vi "Sick Loop.vi"() -> ()   [LabVIEW 2009]
uses:
  <vilib>/Platform/TimedLoop/XDataNode/XDataNode.xnode
  <vilib>/Platform/TimedLoop/XDataNode/loadlvalarms.vi
  <vilib>/Platform/TimedLoop/XDataNode/timing_clust.ctl
  <vilib>/Platform/TimedLoop/XDataNode/nitl_modes.ctl
  <vilib>/Platform/TimedLoop/XDataNode/wakeup.ctl
  TypeDefs/Sensor TypeDefs/FPGA Main ref.ctl
  <vilib>/userDefined/High Color/nirio_resource_hc.ctl
  <vilib>/rvi/interface/nirviOpenFPGA/nirviOpenFPGA.xnode
  FPGA Bitfiles/Q_IGVC_2010.lvproj_FPGA Target_FPGA_MAIN.vi.lvbitx
  <vilib>/FPGAPlugInAG/cRIO-9113/nirviIntfOpen_cRIO-9113.vi
  Functional Global Variables/Actions for FG's.ctl
  UI Comm/Watchdog Dish Labels.ctl
  <vilib>/Platform/TimedLoop/XDataNode/XDNodeRunTimeDep.lvlib
panel:
  in  "SICK Init Complete":bool
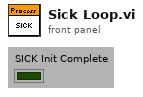
[diagram p1: front panel]
types:
  T1 = typedef "FPGA Main ref.ctl" = refnum<k20>
  T2 = typedef "nirio_resource_hc.ctl" = tag
  T3 = cluster{"signature":u8[], "vi signatures match":bool, "signature register address":u32, "reset register address":u32, "control register address":u32, "interrupt base address":u32, "Bitstream Version":u32, "DMA Configuration":cluster{"Name":string, "Depth":u32, "Write? (Deprecated:Use Implementation)":bool, "Physical Channel":u32, "Base Address":u32, "Data Width":u32, "Data Type":enum32{"Boolean", "I8", "I16", "I32", "I64", "U8", "U16", "U32", "U64", "FXP"}, "FXP Properties":variant, "Write Window Address":u32, "Implementation":enum16{"niFpgaTargetToHost", "niFpgaHostToTarget", "niFpgaPeerToPeerWriter", "niFpgaPeerToPeerReader", "niCoreTargetToHost", "niCoreHostToTarget"}, "Control Set":u32}[], "run when loaded?":bool, "reset register size in bits":u32, "compilation results xml":string}
  T4 = typedef "XDNodeRunTimeDep.lvlib/timing_clust.ctl" = cluster{"Expected End [f-1]":u64, "Actual End [f-1]":u64, "Finished Late? [f-1]":bool, "Expected End [i-1]":u64, "Actual End [i-1]":u64, "Finished Late? [i-1]":bool, "Expected Start [i]":u64, "Actual Start [i]":u64, "Expected Start [f]":u64, "Actual Start [f]":u64, "Source Name":string, "Structure Name":string, "Period":i64, "Deadline":i64, "Offset":i64, "Start":i64, "Priority":i32, "Timeout":i32, "Mode":T5, "Wakeup Reason":T6, "Error":errorcluster, "Source Type":string, "Secondary Source Type":string, "Global End Time":u64, "Global Start Time":u64, "Frame Duration":u64, "Iteration Duration":u64, "Assigned CPU":i32, "I/O Scan Engine Mode":u32}
  T5 = typedef "XDNodeRunTimeDep.lvlib/nitl_modes.ctl" = enum32{"No Change", "Process missed periods, maintain original phase", "Discard missed periods, maintain original phase", "Process missed periods, ignore original phase", "Discard missed periods, ignore original phase"}
  T6 = typedef "XDNodeRunTimeDep.lvlib/wakeup.ctl" = enum32{"Normal", "Aborted", "Asynchronous wakeup", "Timing source error", "Timed loop error", "Timeout"}
  T7 = typedef "SICK Array.ctl" = u16[]
  T8 = typedef "Actions for FG's.ctl" = enum16{"Read", "Write"}
  T9 = typedef "Watchdog Dish Labels.ctl" = enum16{"GPS", "SICK", "Compass", "Cameras", "Motor Controller", "Debug", "RC Receiver"}
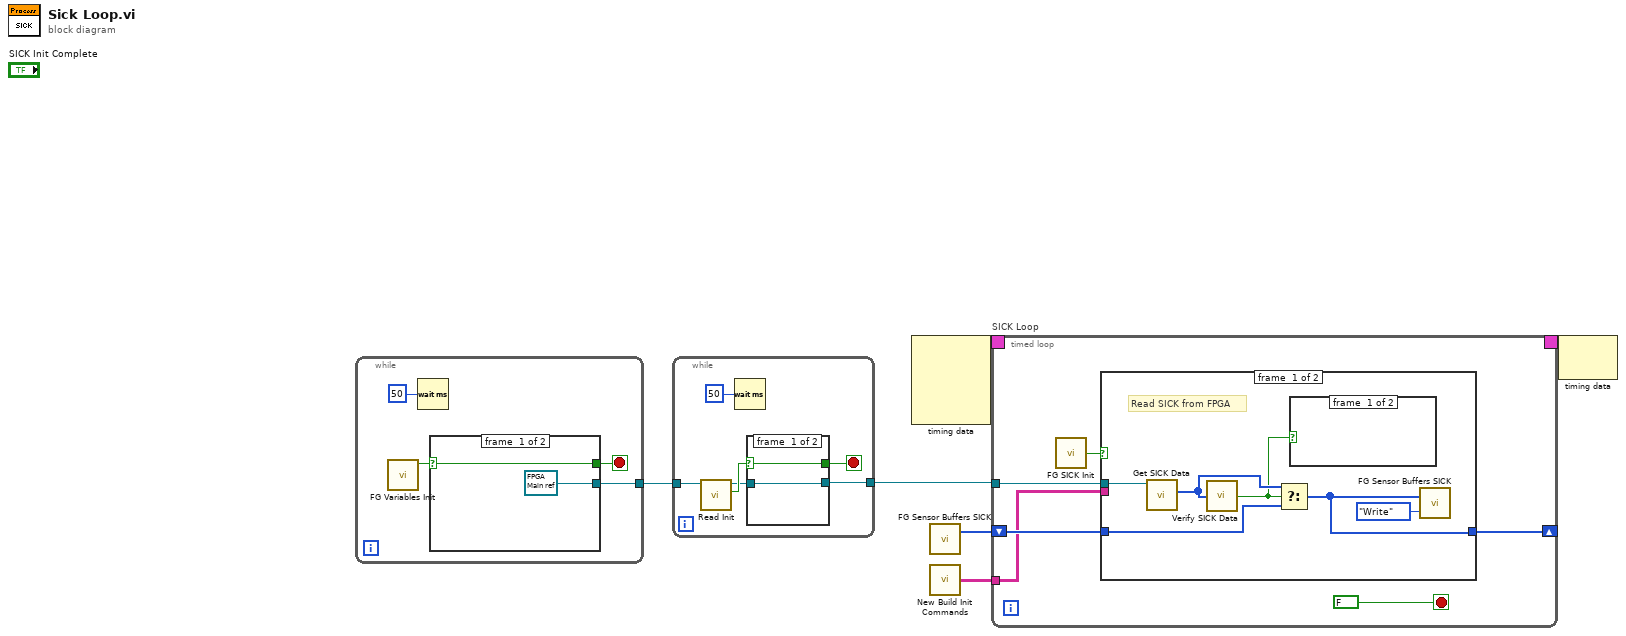
[diagram p0: block diagram]
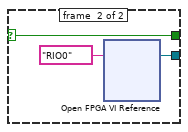
[diagram p2: hidden frame]
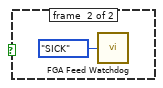
[diagram p4: hidden frame]
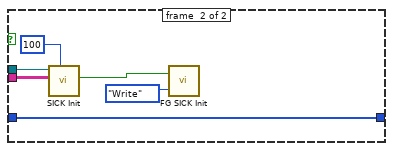
[diagram p5: hidden frame]
diagram:
  n1 = while {
    tunnel: [w8] -> w1
    stop <- w9 stop-if-true
    n2 = call "FG Variables Init.vi"() -> ("Variables Init out"=w10:bool)  [unwired: 11 in]
    n3 = Wait (ms)(milliseconds to wait=u32 50) -> ()  [unwired: 1 out]
    n4 = case shown="True" w10 {
      selector: w10 -> [w12 w15]
      tunnel: [w12 w15] -> w9
      tunnel: [T1 refnum ("FPGA VI Reference out") w13] -> w8
      frame #0 {
      }
      frame #1 {
        n5 = xnode "Open FPGA VI Reference"("resource name"=T2 "RIO0") -> ("FPGA VI Reference Out"=w13:refnum<k20>)  [unwired: 1 in, 1 out]
      }
    }
  }
  n6 = while {
    tunnel: [w31] -> w2
    tunnel: w1 -> [w29]
    stop <- w32 stop-if-true
    n7 = call "Read Init.vi"("FPGA VI Reference in"=w29) -> ("FPGA VI Reference out"=w27:T1, "Init switch"=w28:bool)  [unwired: 7 in, 1 out]
    n8 = Wait (ms)(milliseconds to wait=u32 50) -> ()  [unwired: 1 out]
    n9 = case shown="True" w28 {
      selector: w28 -> [w34 w36]
      tunnel: [w34 w36] -> w32
      tunnel: [w33 w35] -> w31
      tunnel: w27 -> [w33 w35]
      frame #0 {
      }
      frame #1 {
      }
    }
  }
  n10 = node-c288() -> (w6:T4)  [unwired: 4 in]
  n11 = call "FG Sensor Buffers SICK.vi"() -> ("SICK Buffer out"=w4:T7)  [unwired: 3 in]
  n12 = call "New Build Init Commands.vi"() -> ("SICK Commands"=w3:string[][])
  n13 = timed-loop "SICK Loop" {
    timing: w6 -> [_]
    timing-out: [_] -> w5
    tunnel: w2 -> [w41]
    shift-right: [w39] -> _
    shift-left: w4 -> [w40]
    tunnel: w3 -> [w38]
    stop <- FALSE stop-if-true
    n14 = call "FG SICK Init.vi"() -> ("SICK Init out"=w37:bool)  [unwired: 2 in]
    n15 = case shown="True" w37 {
      tunnel: w41 -> [w48 w54]
      tunnel: w40 -> [w46 w55]
      tunnel: [w44 w55] -> w39
      tunnel: w38 -> [_ w53]
      frame #0 {
        # "Read SICK from FPGA"
        n16 = call "Get SICK Data.vi"("FPGA_MAIN ref in"=w48) -> ("SICK Data"=w47:T7)  [unwired: 7 in, 3 out]
        n17 = call "Verify SICK Data.vi"("SICK Data"=w47) -> ("Data OK?"=w43:bool)
        n18 = Select(t=w47, s=w43, f=w46) -> (s? t:f=w44:T7)
        n19 = case shown="True" w43 {
          frame #0 {
          }
          frame #1 {
            n20 = call "FGA Feed Watchdog.vi"("Watchdog Dish"=Watchdog_Dish_Labels."SICK") -> ()  [unwired: 1 out]
          }
        }
        n21 = call "FG Sensor Buffers SICK.vi"("FG Actions (Read)"=Actions_for_FG's."Write" ("FG Actions"), "SICK Buffer in"=w44) -> ()  [unwired: 1 in, 1 out]
      }
      frame #1 {
        n22 = call "SICK Init.vi"("SICK Init Timeout"=100, "SICK Commands"=w53, "FPGA_MAIN ref in"=w54) -> ("Init Success"=w51:bool)  [unwired: 6 in, 2 out]
        n23 = call "FG SICK Init.vi"("FG Action"=Actions_for_FG's."Write", "SICK Init in"=w51) -> ()  [unwired: 1 out]
      }
    }
  }
  n24 = node-c288(w5) -> ()  [unwired: 1 out]
